vi "Teleop.vi"(10 "Match Info":T1={"Autonomous Elapsed Seconds"=0.0, "TeleOp Elapsed Seconds"=0.0, "Disabled Elapsed Seconds"=0.0, "Visited Autonomous"=FALSE, "Visited TeleOp"=FALSE, "Visited Disabled"=FALSE, "Autonomous Settings"={"Autonomous Style"=enum."Independent", "VI Refnum"=refnum}}, 11 "Call Context":T2) -> ()   [LabVIEW 2019]
doc: "This VI is called for each TeleOp packet received from the DS where the robot is not disabled. It is often used to read from the joysticks and update I/O or to update setpoints for timed control loops. It should complete and return within 20 milliseconds or it may miss DS packets."
uses:
  <vilib>/Rock Robotics/WPI/DriverStation/WPI_DriverStationDerivedRobotMode.ctl
  <vilib>/Rock Robotics/WPI/DriverStation/WPI_DriverStationMatch Info.ctl
  <vilib>/Rock Robotics/WPI/Utilities/WPI_GetSetVariantRefNum.vi
  <vilib>/Rock Robotics/Network Tables/NT Write Boolean Array.vi
  <vilib>/Rock Robotics/Network Tables/NT Write Numeric Array.vi
  <vilib>/Rock Robotics/Network Tables/NT Read Boolean.vi
  <vilib>/Rock Robotics/Network Tables/NT Read Number.vi
  <vilib>/Rock Robotics/Network Tables/NT Write Number.vi
panel:
  out "Bottom Limit":bool
  out "Upper Limit":bool
  out "GoDown?":bool
  out "Time":dbl
  out "Throttle":dbl
  out "Sample Slider 0":dbl(slide) scale=0.0..5.0
  out "Sample Boolean 1":bool
  out "Sample Boolean 0":bool
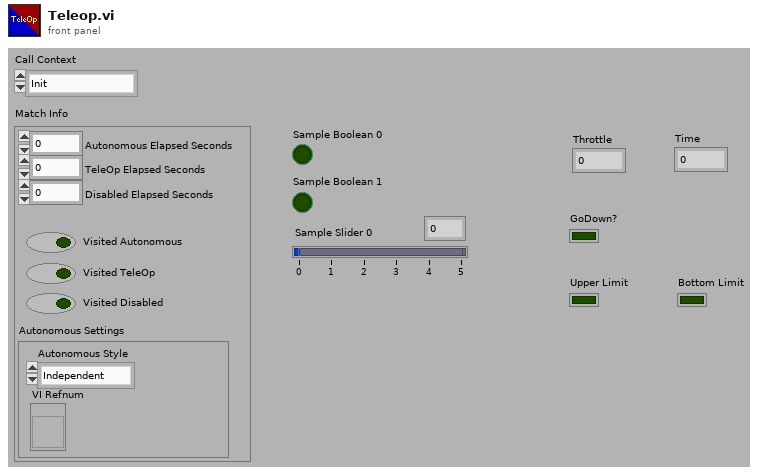
[diagram p1: front panel]
types:
  T1 = typedef "WPI_DriverStationMatch Info.ctl" = cluster{"Autonomous Elapsed Seconds":dbl, "TeleOp Elapsed Seconds":dbl, "Disabled Elapsed Seconds":dbl, "Visited Autonomous":bool, "Visited TeleOp":bool, "Visited Disabled":bool, "Autonomous Settings":cluster{"Autonomous Style":enum16{"Iterative", "Independent"}, "VI Refnum":refnum<vi>}}
  T2 = typedef "WPI_DriverStationDerivedRobotMode.ctl" = enum16{"Init", "Execute", "Stop"}
  T3 = typedef "WPI_RobotDriveDevRef.ctl" = cluster{"DevStatus":errorcluster, "Motors[]":T4[], "Square Inputs":bool, "Max Output":dbl}
  T4 = typedef "WPI_MotorControlDeviceRef.ctl" = cluster{"DeviceStatus":errorcluster, "Type":T5, "PWM":cluster{"PWM Channel":T6, "DeadBand":T7}, "CAN":cluster{"Device Number":u8, "SetOutput VI Ref":variant, "GetOutput VI Ref":variant, "Enable VI Ref":variant, "Disable VI Ref":variant, "Data":variant}, "Invert":bool, "DIO PWM":cluster{"PWM \"Enable\" Channel":T6, "DIOChannel":T8, "PWM Rate":dbl}}
  T5 = typedef "WPI_MotorControlType.ctl" = enum16{"PWM", "CAN", "DIO PWM"}
  T6 = typedef "FPGA_DIOPWMChannel.ctl" = enum8{"PWM 0", "PWM 1", "PWM 2", "PWM 3", "PWM 4", "PWM 5", "PWM 6", "PWM 7", "PWM 8", "PWM 9", "PWM MXP 0", "PWM MXP 1", "PWM MXP 2", "PWM MXP 3", "PWM MXP 4", "PWM MXP 5", "PWM MXP 6", "PWM MXP 7", "PWM MXP 8", "PWM MXP 9", "Invalid"}
  T7 = typedef "WPI_PWMDeadband.ctl" = cluster{"Name":string, "maxPositivePwm":i32, "minPositivePwm":i32, "centerPwm":i32, "maxNegativePwm":i32, "minNegativePwm":i32, "angularRange":u16}
  T8 = typedef "FPGA_DIOChannel.ctl" = enum8{"DIO 0", "DIO 1", "DIO 2", "DIO 3", "DIO 4", "DIO 5", "DIO 6", "DIO 7", "DIO 8", "DIO 9", "DIO MXP 0", "DIO MXP 1", "DIO MXP 2", "DIO MXP 3", "DIO MXP 4", "DIO MXP 5", "DIO MXP 6", "DIO MXP 7", "DIO MXP 8", "DIO MXP 9", "DIO MXP 10", "DIO MXP 11", "DIO MXP 12", "DIO MXP 13", "DIO MXP 14", "DIO MXP 15", "SPI Port CS1", "SPI Port CS2", "SPI Port CS3", "SPI Port MISO", "SPI Port MOSI", "Invalid"}
  T9 = typedef "WPI_JoystickDevRef.ctl" = cluster{"Device":T10}
  T10 = typedef "WPI_JoystickDeviceEnum.ctl" = enum16{"USB 0", "USB 1", "USB 2", "USB 3", "USB 4", "USB 5"}
  T11 = typedef "WPI_DigitalOutputDevRef.ctl" = cluster{"DIO Channel":T8, "DevStatus":errorcluster}
  T12 = typedef "WPI_SwitchDevRef.ctl" = cluster{"DevStatus":errorcluster, "DIO Channel":T8, "CntIndex":T13, "Normally Closed":bool}
  T13 = typedef "FPGA_CounterCtrSystemIndex.ctl" = enum8{"Ctr 0", "Ctr 1", "Ctr 2", "Ctr 3", "Ctr 4", "Ctr 5", "Ctr 6", "Ctr 7", "Invalid"}
  T14 = typedef "WPI_GyroDevRef.ctl" = cluster{"DevStatus":errorcluster, "Analog Channel":T15, "Gain (VoltsPerDegree/Second)":dbl, "Gyro Type":enum16{"Analog", "XRS450"}, "Handle":i32, "SPI Bus":T16, "Device Found":bool, "Sample Rate":dbl, "Calibrate On Open":bool, "Offset":dbl}
  T15 = typedef "FPGA_AIChannel.ctl" = enum8{"AI 0", "AI 1", "AI 2", "AI 3", "AI MXP 0", "AI MXP 1", "AI MXP 2", "AI MXP 3", "Invalid"}
  T16 = typedef "spi_bus.ctl" = enum16{"SPI On-Board, CS0", "SPI On-Board, CS1", "SPI On-Board, CS2", "SPI On-Board, CS3", "SPI MXP", "Invalid"}
  T17 = typedef "WPI_EncoderDevRef.ctl" = cluster{"DevStatus":errorcluster, "EncoderIndex":T18, "CounterIndex":T13, "DistancePerCount":dbl, "Decoding Type":T19}
  T18 = typedef "FPGA_EncoderIdx.ctl" = enum8{"Enc 0", "Enc 1", "Enc 2", "Enc 3", "Enc 4", "Enc 5", "Enc 6", "Enc 7", "Invalid"}
  T19 = typedef "WPI_EncoderType.ctl" = enum16{"1x", "2x", "4x"}
  T20 = typedef "WPI_AnalogChannelDevRef.ctl" = cluster{"DevStatus":errorcluster, "Analog Channel":T15}
  T21 = typedef "WPI_AccelerometerDevRef.ctl" = cluster{"DevStatus":errorcluster, "Scaling":T22, "Analog Channels":T23, "I2C Bus":T24, "SPI Bus":T16, "Accel Range":T25, "ADXL Axes":T26, "Handle":i32, "Device Address":u8, "Accel Type":enum16{"Analog", "ADXL345 I2C", "ADXL345 SPI", "Internal", "ADXL362 SPI"}}
  T22 = typedef "WPI_AccelerometerScaling.ctl" = cluster{"Gain (VoltsPerG)":dbl, "Center Voltage":dbl}
  T23 = typedef "WPI_AccelerometerAnalogChannels.ctl" = cluster{"X-Axis":T15, "Y-Axis":T15, "Z-Axis":T15}
  T24 = typedef "i2c_bus.ctl" = enum16{"I2C On-Board", "I2C MXP", "Invalid"}
  T25 = typedef "ADXL345 Range.ctl" = u8
  T26 = typedef "WPI_AccelerometerADXL345 Axes.ctl" = cluster{"X-Axis":bool, "Y-Axis":bool, "Z-Axis":bool}
  T27 = cluster{"X-Axis":dbl, "Y-Axis":dbl, "Z-Axis":dbl}
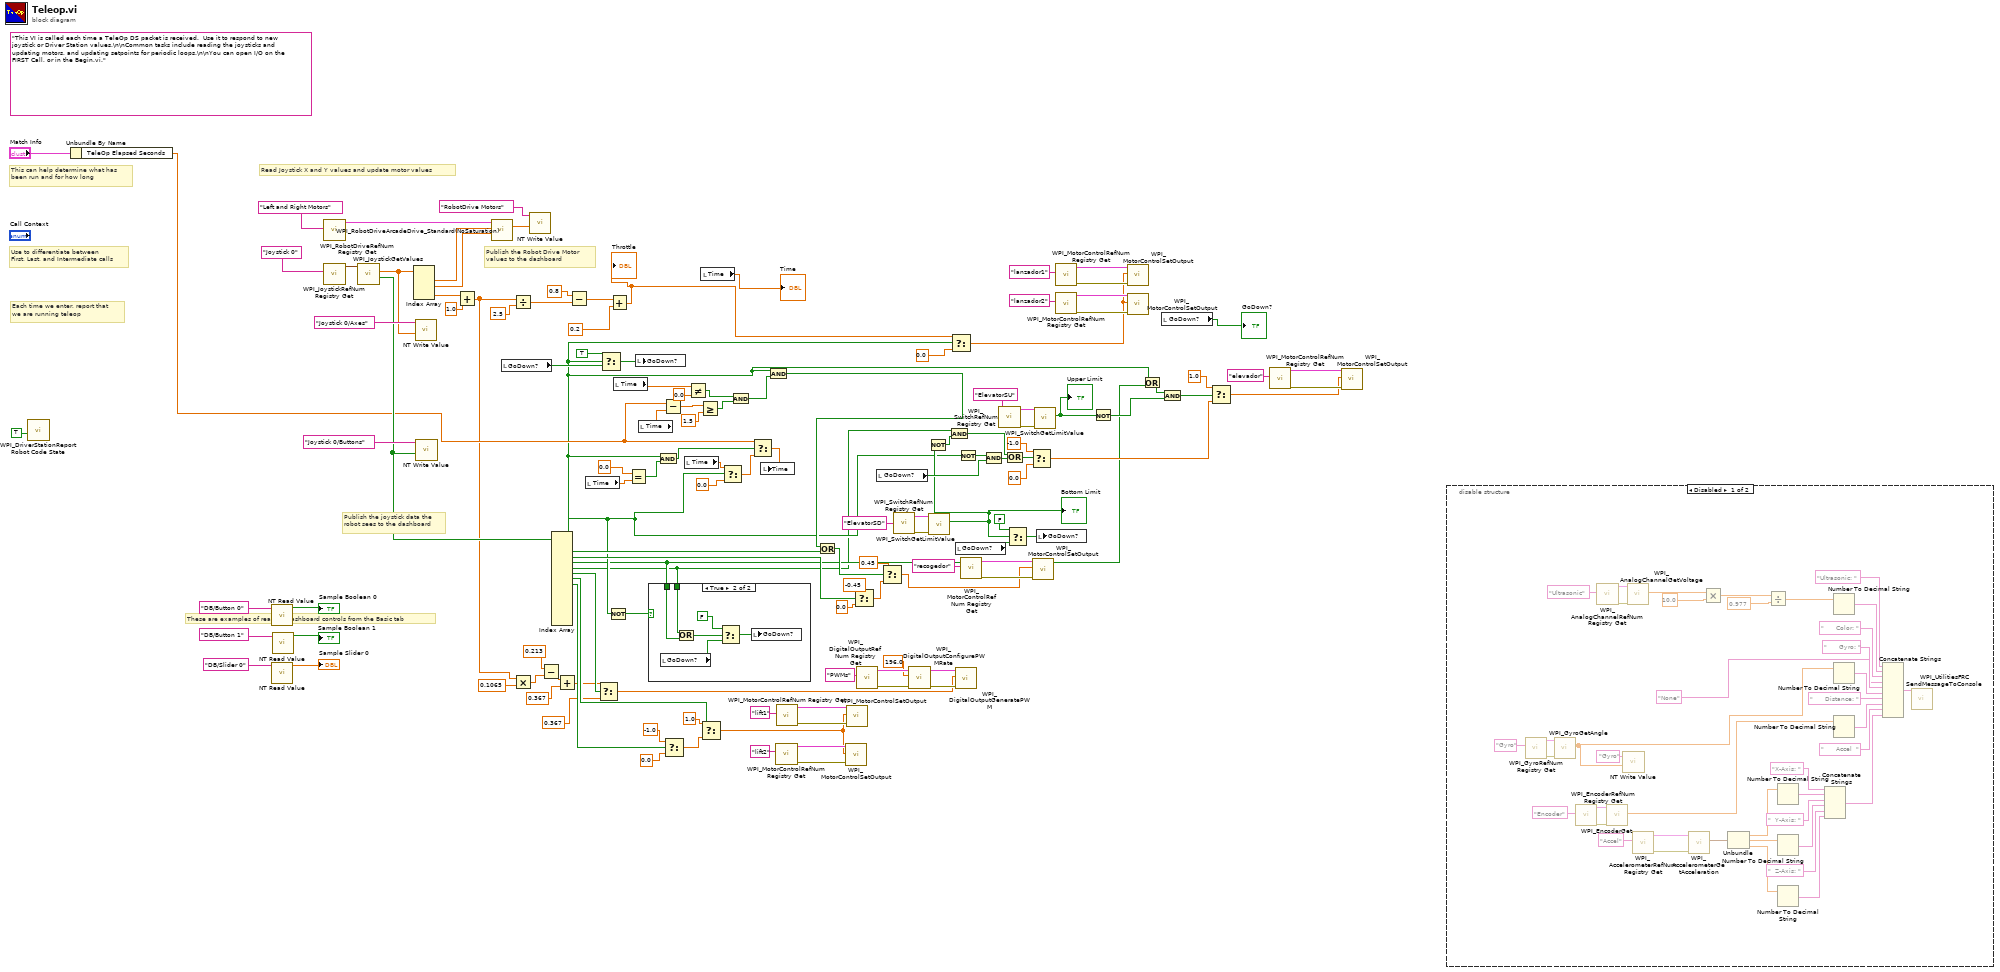
[diagram p0: block diagram]
diagram:
  (unwired) "This VI is called each time a TeleOp DS packet is received.  Use it to respond to new joystick or Driver Station values.\n\nCommon tasks include reading the joysticks and updating motors, and updating setpoints for periodic loops.\n\nYou can open I/O on the FIRST Call, or in the Begin.vi."
  # "These are examples of reading dashboard controls from the Basic tab"
  # "Publish the Robot Drive Motor\nvalues to the dashboard"
  # "Publish the joystick data the\nrobot sees to the dashboard"
  # "Each time we enter, report that\nwe are running teleop"
  # "Use to differentiate between\nFirst, Last, and Intermediate calls"
  # "This can help determine what has\nbeen run and for how long"
  # "Read Joystick X and Y values and update motor values"
  n1 = call <vilib>:"WPI_DriverStationReport Robot Code State.vi"("TeleOp"=TRUE ("Autonomous")) -> ()  [unwired: 10 in, 1 out]
  n2 = Unbundle By Name("Match Info") -> ("TeleOp Elapsed Seconds"=w68:dbl)
  n3 = call-poly <vilib>:"NT Read Value.vi"("Name"="DB/Button 0" ("refnum name")) -> ("Boolean"=→"Sample Boolean 0":bool)  [unwired: 9 in, 1 out]
  n4 = call-poly <vilib>:"NT Read Value.vi"("Name"="DB/Slider 0" ("refnum name")) -> ("Numeric"=→"Sample Slider 0":dbl)  [unwired: 9 in, 1 out]
  n5 = call-poly <vilib>:"NT Read Value.vi"("Name"="DB/Button 1" ("refnum name")) -> ("Boolean"=→"Sample Boolean 1":bool)  [unwired: 9 in, 1 out]
  n6 = call <vilib>:"WPI_RobotDriveRefNum Registry Get.vi"("refnum name"="Left and Right Motors") -> ("RobotDriveDevRef"=w128:T3)  [unwired: 1 in, 9 out]
  n7 = call <vilib>:"WPI_JoystickRefNum Registry Get.vi"("refnum name"="Joystick 0") -> ("JoystickDevRef"=w125:T9)  [unwired: 1 in, 9 out]
  n8 = call <vilib>:"WPI_JoystickGetValues.vi"("JoystickDevRef"=w125) -> ("Buttons"=w112:bool[], "Axes"=w121:dbl[])  [unwired: 6 in, 3 out]
  n9 = Index Array(array=w121) -> (element #1=w127:dbl, element #2=w41:dbl, element #4=w21:dbl)  [unwired: 4 in, 1 out]
  n10 = call-poly <vilib>:"NT Write Value.vi"("Numeric Array"=w121, "Name"="Joystick 0/Axes") -> ()  [unwired: 9 in, 1 out]
  n11 = call-poly <vilib>:"NT Write Value.vi"("Boolean Array"=w112, "Name"="Joystick 0/Buttons") -> ()  [unwired: 9 in, 1 out]
  n12 = Add(x=w21, y=1.0) -> (x+y=w2:dbl)
  n13 = call <vilib>:"WPI_RobotDriveArcadeDrive_Standard(NoSaturation).vi"("Y axis value"=w41, "X axis value"=w127, "RobotDriveDevRef"=w128) -> ("Motor Values"=w114:dbl[])  [unwired: 1 in, 7 out]
  n14 = local read "GoDown?"() -> (w51:bool)
  n15 = Divide(x=w2, y=2.5) -> (x/y=w24:dbl)
  n16 = Multiply(x=w2, y=0.1065) -> (x*y=w7:dbl)
  n17 = call-poly <vilib>:"NT Write Value.vi"("Numeric Array"=w114, "Name"="RobotDrive Motors") -> ()  [unwired: 9 in, 1 out]
  n18 = Subtract(x=0.213, y=w7) -> (x-y=w5:dbl)
  n19 = Index Array(array=w112) -> (element #1=w28:bool, element #2=w56:bool, element #3=w110:bool, element #4=w19:bool, element #5=w18:bool, element #6=w10:bool, element #7=w17:bool, element #8=w16:bool)  [unwired: 15 in, 7 out]
  n20 = Add(x=w5, y=0.367) -> (x+y=w3:dbl)
  n21 = Subtract(x=0.8, y=w24) -> (x-y=w23:dbl)
  n22 = local read "Time"() -> (w85:dbl)
  n23 = Select(t=w3, s=w10, f=0.367) -> (s? t:f=w9:dbl)
  n24 = Select(t=TRUE, s=w28, f=w51) -> (s? t:f=w52:bool)
  n25 = Not(x=w28) -> (.not. x?=w29:bool)
  n26 = Add(x=w23, y=0.2) -> (x+y=w20:dbl)
  "Throttle" <- w20
  n27 = local read "Time"() -> (w62:dbl)
  n28 = Equal?(x=0.0, y=w85) -> (x = y?=w86:bool)
  n29 = local write "GoDown?"(w52) -> ()
  n30 = local read "Time"() -> (w67:dbl)
  n31 = case shown="True" w29 {
    tunnel: w18 -> [_ w135]
    tunnel: w19 -> [_ w134]
    frame False {
    }
    frame True {
      n32 = local read "GoDown?"() -> (w131:bool)
      n33 = Or(x=w135, y=w134) -> (x .or. y?=w136:bool)
      n34 = Select(t=FALSE, s=w136, f=w131) -> (s? t:f=w132:bool)
      n35 = local write "GoDown?"(w132) -> ()
    }
  }
  n36 = And(x=w28, y=w86) -> (x .and. y?=w87:bool)
  n37 = Subtract(x=w68, y=w67) -> (x-y=w66:dbl)
  n38 = Select(t=-1.0, s=w16, f=0.0) -> (s? t:f=w102:dbl)
  n39 = local read "Time"() -> (w59:dbl)
  n40 = Not Equal?(x=w62, y=0.0) -> (x != y?=w63:bool)
  n41 = Greater Or Equal?(x=w66, y=1.5) -> (x >= y?=w64:bool)
  n42 = Select(t=1.0, s=w17, f=w102) -> (s? t:f=w44:dbl)
  n43 = local read "Time"() -> (→"Time":dbl)
  n44 = Select(t=w59, s=w28, f=0.0) -> (s? t:f=w57:dbl)
  n45 = And(x=w63, y=w64) -> (x .and. y?=w60:bool)
  n46 = Select(t=w68, s=w87, f=w57) -> (s? t:f=w88:dbl)
  n47 = local write "Time"(w88) -> ()
  n48 = And(x=w28, y=w60) -> (x .and. y?=w54:bool)
  n49 = call <vilib>:"WPI_MotorControlRefNum Registry Get.vi"("refnum name"="lift2") -> ("error out"=w47:errorcluster, "MotorControlDevRef"=w46:T4)  [unwired: 9 in]
  n50 = call <vilib>:"WPI_MotorControlRefNum Registry Get.vi"("refnum name"="lift1") -> ("error out"=w100:errorcluster, "MotorControlDevRef"=w98:T4)  [unwired: 9 in]
  n51 = Or(x=w54, y=w56) -> (x .or. y?=w55:bool)
  n52 = call <vilib>:"WPI_MotorControlSetOutput.vi"("error in (no error)"=w47, "Output"=w44, "MotorControlDevRef"=w46) -> ()  [unwired: 6 in, 3 out]
  n53 = call <vilib>:"WPI_MotorControlSetOutput.vi"("error in (no error)"=w100, "Output"=w44, "MotorControlDevRef"=w98) -> ()  [unwired: 6 in, 3 out]
  n54 = Select(t=-0.45, s=w110, f=0.0) -> (s? t:f=w107:dbl)
  n55 = call <vilib>:"WPI_DigitalOutputRefNum Registry Get.vi"("refnum name"="PWMs") -> ("error out"=w13:errorcluster, "DigitalOutputDevRef"=w15:T11)  [unwired: 9 in]
  n56 = local read "GoDown?"() -> (w50:bool)
  n57 = Select(t=0.45, s=w55, f=w107) -> (s? t:f=w103:dbl)
  n58 = call <vilib>:"WPI_SwitchRefNum Registry Get.vi"("refnum name"="ElevatorSD") -> ("error out"=w73:errorcluster, "SwitchDevRef"=w74:T12)  [unwired: 9 in]
  n59 = call <vilib>:"WPI_DigitalOutputConfigurePWMRate.vi"("error in (no error)"=w13, "PWM Rate (Hz)"=sgl 196.0) -> ("error out"=w14:errorcluster)  [unwired: 8 in, 1 out]
  n60 = call <vilib>:"WPI_SwitchGetLimitValue.vi"("error in (no error)"=w73, "SwitchDevRef"=w74) -> ("Switch Pressed"=w37:bool)  [unwired: 7 in, 2 out]
  "Bottom Limit" <- w37
  n61 = Not(x=w37) -> (.not. x?=w36:bool)
  n62 = And(x=w18, y=w36) -> (x .and. y?=w35:bool)
  n63 = Select(t=w20, s=w28, f=0.0) -> (s? t:f=w83:dbl)
  n64 = local read "GoDown?"() -> (w31:bool)
  n65 = call <vilib>:"WPI_DigitalOutputGeneratePWM.vi"("error in (no error)"=w14, "PWM Duty Cycle"=w9, "DigitalOutputDevRef"=w15) -> ()  [unwired: 7 in, 2 out]
  n66 = Not(x=w28) -> (.not. x?=w38:bool)
  n67 = call <vilib>:"WPI_MotorControlRefNum Registry Get.vi"("refnum name"="recogedor") -> ("error out"=w104:errorcluster, "MotorControlDevRef"=w106:T4)  [unwired: 9 in]
  n68 = And(x=w38, y=w50) -> (x .and. y?=w34:bool)
  n69 = call <vilib>:"WPI_SwitchRefNum Registry Get.vi"("refnum name"="ElevatorSU") -> ("error out"=w80:errorcluster, "SwitchDevRef"=w81:T12)  [unwired: 9 in]
  n70 = Or(x=w35, y=w34) -> (x .or. y?=w33:bool)
  n71 = Select(t=FALSE, s=w37, f=w31) -> (s? t:f=w30:bool)
  n72 = Select(t=-1.0, s=w33, f=0.0) -> (s? t:f=w39:dbl)
  n73 = call <vilib>:"WPI_MotorControlSetOutput.vi"("error in (no error)"=w104, "Output"=w103, "MotorControlDevRef"=w106) -> ()  [unwired: 6 in, 3 out]
  n74 = call <vilib>:"WPI_SwitchGetLimitValue.vi"("error in (no error)"=w80, "SwitchDevRef"=w81) -> ("Switch Pressed"=w48:bool)  [unwired: 7 in, 2 out]
  "Upper Limit" <- w48
  n75 = local write "GoDown?"(w30) -> ()
  n76 = call <vilib>:"WPI_MotorControlRefNum Registry Get.vi"("refnum name"="lanzador1") -> ("error out"=w90:errorcluster, "MotorControlDevRef"=w92:T4)  [unwired: 9 in]
  n77 = call <vilib>:"WPI_MotorControlRefNum Registry Get.vi"("refnum name"="lanzador2") -> ("error out"=w93:errorcluster, "MotorControlDevRef"=w95:T4)  [unwired: 9 in]
  n78 = Not(x=w48) -> (.not. x?=w71:bool)
  n79 = call <vilib>:"WPI_MotorControlSetOutput.vi"("error in (no error)"=w90, "Output"=w83, "MotorControlDevRef"=w92) -> ()  [unwired: 6 in, 3 out]
  n80 = call <vilib>:"WPI_MotorControlSetOutput.vi"("error in (no error)"=w93, "Output"=w83, "MotorControlDevRef"=w95) -> ()  [unwired: 6 in, 3 out]
  n81 = Or(x=w28, y=w19) -> (x .or. y?=w40:bool)
  n82 = local read "GoDown?"() -> (→"GoDown?":bool)
  n83 = And(x=w40, y=w71) -> (x .and. y?=w78:bool)
  n84 = Select(t=1.0, s=w78, f=w39) -> (s? t:f=w49:dbl)
  n85 = call <vilib>:"WPI_MotorControlRefNum Registry Get.vi"("refnum name"="elevador") -> ("error out"=w75:errorcluster, "MotorControlDevRef"=w77:T4)  [unwired: 9 in]
  n86 = call <vilib>:"WPI_MotorControlSetOutput.vi"("error in (no error)"=w75, "Output"=w49, "MotorControlDevRef"=w77) -> ()  [unwired: 6 in, 3 out]
  n87 = disable-structure shown="Disabled" {
    frame Disabled {
      n88 = call <vilib>:"WPI_GyroRefNum Registry Get.vi"("refnum name"="Gyro") -> ("error out"=w164:errorcluster, "GyroDevRef"=w165:T14)  [unwired: 9 in]
      n89 = call <vilib>:"WPI_GyroGetAngle.vi"("error in"=w164, "GyroDevRef"=w165) -> ("Angle"=w138:dbl)  [unwired: 5 in, 4 out]
      n90 = call <vilib>:"WPI_EncoderRefNum Registry Get.vi"("refnum name"="Encoder") -> ("error out"=w159:errorcluster, "EncoderDevRef"=w160:T17)  [unwired: 9 in]
      n91 = call <vilib>:"WPI_AnalogChannelRefNum Registry Get.vi"("refnum name"="Ultrasonic") -> ("error out"=w176:errorcluster, "AIDeviceRef"=w177:T20)  [unwired: 9 in]
      n92 = call <vilib>:"WPI_EncoderGet.vi"("error in (no error)"=w159, "EncoderDevRef"=w160) -> ("Distance"=w157:dbl)  [unwired: 4 in, 5 out]
      n93 = call-poly <vilib>:"NT Write Value.vi"("Numeric"=w138, "Name"="Gyro") -> ()  [unwired: 9 in, 1 out]
      n94 = call <vilib>:"WPI_AnalogChannelGetVoltage.vi"("error in (no error)"=w176, "AIDeviceRef"=w177) -> ("Voltage"=w174:dbl)  [unwired: 7 in, 2 out]
      n95 = call <vilib>:"WPI_AccelerometerRefNum Registry Get.vi"("refnum name"="Accel") -> ("error out"=w152:errorcluster, "AccelerometerDevRef"=w153:T21)  [unwired: 9 in]
      n96 = call <vilib>:"WPI_AccelerometerGetAcceleration.vi"("error in"=w152, "AccelerometerDevRef"=w153) -> ("Accelerations"=w151:T27)  [unwired: 7 in, 2 out]
      n97 = Multiply(x=w174, y=10.0) -> (x*y=w172:dbl)
      n98 = Unbundle(w151) -> ("X-Axis"=w148:dbl, "Y-Axis"=w146:dbl, "Z-Axis"=w145:dbl)
      n99 = Divide(x=w172, y=0.977) -> (x/y=w170:dbl)
      n100 = Number To Decimal String(number=w148) -> (decimal integer string=w147:string)  [unwired: 1 in]
      n101 = Number To Decimal String(number=w146) -> (decimal integer string=w144:string)  [unwired: 1 in]
      n102 = Number To Decimal String(number=w145) -> (decimal integer string=w143:string)  [unwired: 1 in]
      n103 = Concatenate Strings("X-Axis: " ("string"), w147, "  Y-Axis: " ("string"), w144, "  Z-Axis: " ("string"), w143) -> (w140:string)
      n104 = Number To Decimal String(number=w170) -> (decimal integer string=w168:string)  [unwired: 1 in]
      n105 = Number To Decimal String(number=w138) -> (decimal integer string=w162:string)  [unwired: 1 in]
      n106 = Number To Decimal String(number=w157) -> (decimal integer string=w155:string)  [unwired: 1 in]
      n107 = Concatenate Strings("Ultrasonic: " ("string"), w168, "      Color: " ("string"), "None" ("string"), "      Gyro: " ("string"), w162, "      Distance: " ("string"), w155, "      Accel  " ("string"), w140) -> (w161:string)
      n108 = call <vilib>:"WPI_UtilitiesFRC SendMessageToConsole.vi"("Message"=w161) -> ()  [unwired: 14 in, 1 out]
    }
    frame Enabled {
    }
  }
